vi "Database Update.vi"() -> ()   [LabVIEW 2023]
doc: "This example shows how you can update information in a table. Select one of the names in the ring control and enter a new phone number. Click the Change button to complete the update and display the current data in the table."
uses:
  <vilib>/addons/database/Connection.llb/DB Tools Open Connec (Path).vi
  <vilib>/addons/database/_DB Variant To Data/Database Variant To Data.xnode
  <vilib>/addons/database/NI_Database_API.lvlib
panel:
  out "Final Data":string[][](array[string])
  out "Initial Data":string[][](array[string])
  in  "change":bool
  in  "New phone number":string
  in  "Name":u16(ring) items=["Joe Smith", "Greg Myers", "Steve Jones", "Anne Harvey"]
  # "Overview: Demonstrates how to update data in a table in a database.\nRequirements: Database Connectivity Toolkit\nInstructions:\n1. Run the VI.\n2. Specify a Name in the ring.\n3. Specify a New phone number for the selected person.\n4. Click Change to change the phone number of the selected person. The Final Data table will display the updated information."
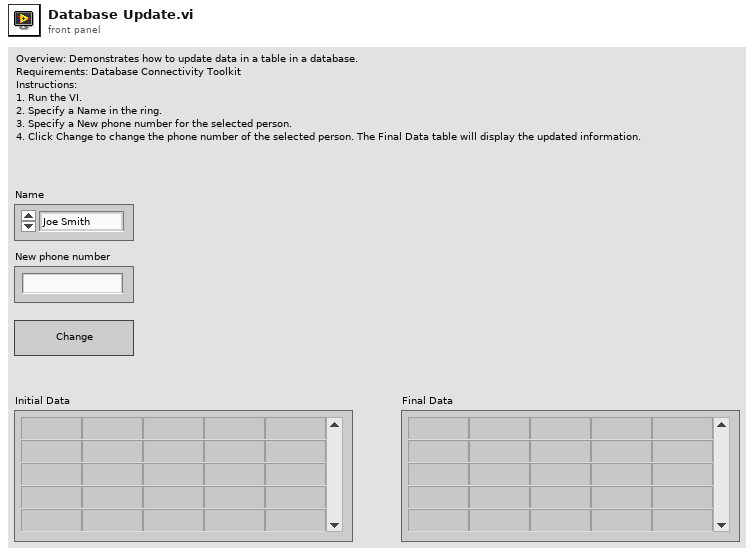
[diagram p1: front panel]
types:
  T1 = typedef "NI_Database_API.lvlib/Conn ObjectReference.ctl" = refnum<k1>
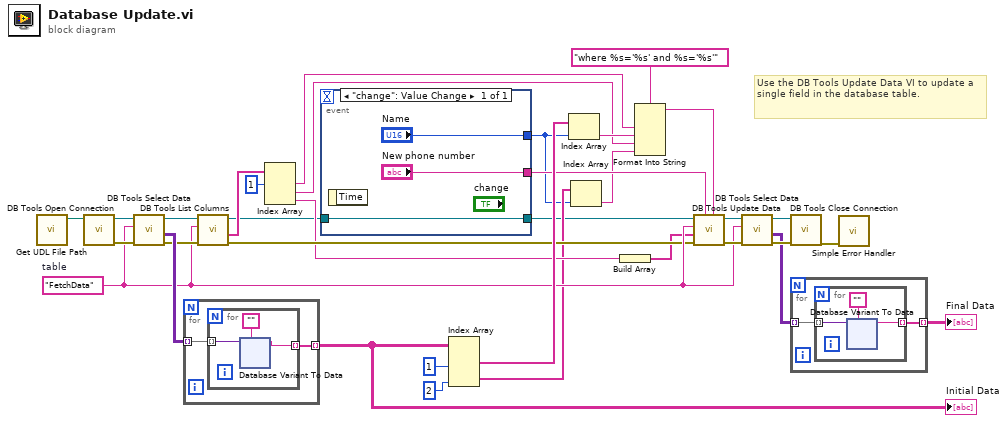
[diagram p0: block diagram]
diagram:
  w19 = "FetchData"  # table
  # "Use the DB Tools Update Data VI to update a single field in the database table."
  n1 = call "Get UDL File Path.vi"() -> ("UDL file path"=w32:path)  [unwired: 11 in]
  n2 = call-poly <vilib>:"DB Tools Open Connection.vi"("connection information"=w32) -> ("error out"=w31:errorcluster, "connection reference"=w33:T1)  [unwired: 7 in]
  n3 = call <vilib>:"DB Tools Select Data.vi"("error in (no error)"=w31, "table"=w19, "connection reference"=w33) -> ("error out"=w20:errorcluster, "data"=w34:variant[][], "connection reference out"=w21:T1)  [unwired: 3 in]
  n4 = for {
    tunnel: w34 -> [w36] mode=indexing
    tunnel: [w35] -> w14 mode=indexing
    n5 = for {
      tunnel: w36 -> [w38] mode=indexing
      tunnel: [w37] -> w35 mode=indexing
      n6 = xnode "Database Variant To Data"("database variant"=w38, "type"="") -> ("data"=w37:string)  [unwired: 1 in, 1 out]
    }
  }
  "Initial Data" <- w14
  n7 = call <vilib>:"DB Tools List Columns.vi"("error in (no error)"=w20, "table"=w19, "connection reference"=w21) -> ("error out"=w16:errorcluster, "columns"=w17:string[], "connection reference out"=w2:T1)  [unwired: 1 in, 1 out]
  n8 = Index Array(array=w17, index #1=1 ("disabled index (col)")) -> (element #1=w7:string, element #2=w5:string, element #3=w11:string)  [unwired: 2 in]
  n9 = event shown="[0] \"change\": Value Change" {
    selector: _ -> [_]
    dyn-events: _ -> [_]
    timeout: _ -> [_]
    tunnel: ["New phone number"] -> w12
    tunnel: ["Name"] -> w9
    tunnel: w2 -> [w72]
    tunnel: [w72] -> w1
    event "change": Value Change {
      n10 = event-data() -> ()  [unwired: 1 in, 1 out]
    }
  }
  n11 = Index Array(array=w14, index (col) #1=1 ("disabled index (col)"), index (col) #2=2 ("index (col)")) -> (element #1=w22:string[], element #2=w10:string[])  [unwired: 2 in]
  n12 = Index Array(array=w22, index=w9) -> (element=w6:string)
  n13 = Index Array(array=w10, index=w9) -> (element=w4:string)
  n14 = Build Array(w11) -> (w15:string[])
  n15 = Format Into String(format string="where %s='%s' and %s='%s'", w7, w6, w5, w4) -> (resulting string=w3:string)  [unwired: 2 in, 1 out]
  n16 = call <vilib>:"DB Tools Update Data.vi"("condition"=w3, "data"=w12, "error in (no error)"=w16, "columns"=w15, "table"=w19, "connection reference"=w1) -> ("error out"=w27:errorcluster, "connection reference out"=w28:T1)  [unwired: 4 in]
  n17 = call <vilib>:"DB Tools Select Data.vi"("error in (no error)"=w27, "table"=w19, "connection reference"=w28) -> ("error out"=w25:errorcluster, "data"=w24:variant[][], "connection reference out"=w26:T1)  [unwired: 3 in]
  n18 = call <vilib>:"DB Tools Close Connection.vi"("error in (no error)"=w25, "connection reference"=w26) -> ("error out"=w23:errorcluster)  [unwired: 5 in]
  n19 = for {
    tunnel: w24 -> [w76] mode=indexing
    tunnel: [w75] -> w13 mode=indexing
    n20 = for {
      tunnel: w76 -> [w78] mode=indexing
      tunnel: [w77] -> w75 mode=indexing
      n21 = xnode "Database Variant To Data"("database variant"=w78, "type"="") -> ("data"=w77:string)  [unwired: 1 in, 1 out]
    }
  }
  "Final Data" <- w13
  n22 = call <vilib>:"Simple Error Handler.vi"("error in (no error)"=w23) -> ()  [unwired: 4 in, 5 out]
